vi "MU Calibration Get Nonius Track Offset Table.vi"(8 "error in (no error)":errorcluster, 11 "CalibrationHandle":T1) -> (0 "error out (no error)":errorcluster, 3 "noniusTrackOffsetTable":cluster{"spoBase":i8, "spoN":i8[]})   [LabVIEW 2017, in "MU_3SL_interface.lvlib"]
uses:
  MU_3SL_interface.lvlib
  handles/CalibrationHandle.ctl
  lib/MU_3SL_interface.dll
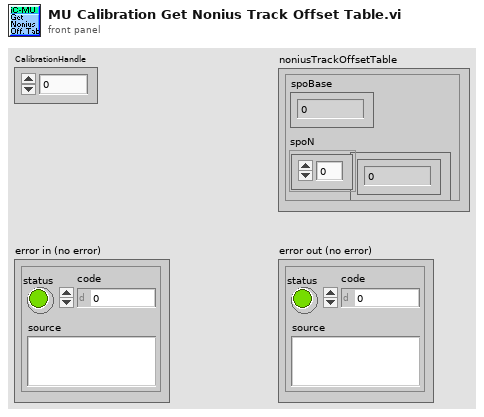
[diagram p1: front panel]
types:
  T1 = typedef "MU_3SL_interface.lvlib/CalibrationHandle.ctl" = u64
  T2 = cluster{"[0]":i8, "[1]":i8, "[2]":i8, "[3]":i8, "[4]":i8, "[5]":i8, "[6]":i8, "[7]":i8, "[8]":i8, "[9]":i8, "[10]":i8, "[11]":i8, "[12]":i8, "[13]":i8, "[14]":i8, "[15]":i8, "[16]":i8}
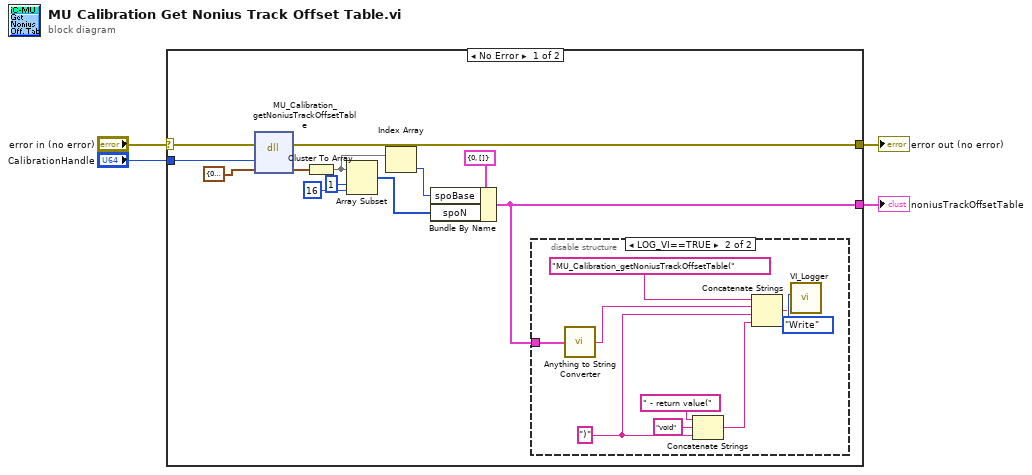
[diagram p0: block diagram]
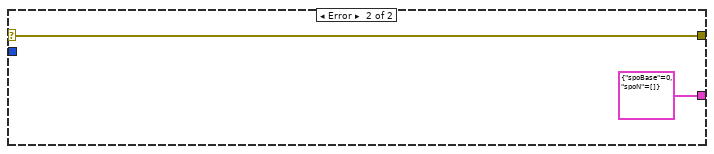
[diagram p3: hidden frame]
diagram:
  n1 = case shown="No Error" "error in (no error)" {
    selector: "error in (no error)" -> [w16 w27]
    tunnel: [w14 w27] -> w4
    tunnel: "CalibrationHandle" -> [w15 _]
    tunnel: [w5 cluster{"spoBase":i8, "spoN":i8[]} {"spoBase"=0, "spoN"=[]} ("optimizedNoniusTrackOffsetTable")] -> w2
    frame No Error {
      n2 = dll-call lib="C:/Users/bes/AppData/Roaming/work/mu_9so/icsubmodules/soft_mu_3sl_master/lv_interface/lib/MU_3SL_interface**.*" fn="MU_Calibration_getNoniusTrackOffsetTable"(error in=w16, "CalibrationHandle"=w15, "noniusTrackOffsetTable"=T2 {"[0]"=0, "[1]"=0, "[2]"=0, "[3]"=0, "[4]"=0, "[5]"=0, "[6]"=0, "[7]"=0, "[8]"=0, "[9]"=0, "[10]"=0, "[11]"=0, "[12]"=0, "[13]"=0, "[14]"=0, "[15]"=0, "[16]"=0}) -> (error out=w14:errorcluster, "noniusTrackOffsetTable"=w8:T2)  [unwired: 4 in, 1 out]
      n3 = Cluster To Array(cluster=w8) -> (array=w11:i8[])
      n4 = Array Subset(array=w11, index=1, length=16) -> (w9:i8[])
      n5 = Index Array(array=w11) -> (element=w10:i8)  [unwired: 1 in]
      n6 = Bundle By Name(cluster=cluster{"spoBase":i8, "spoN":i8[]} {"spoBase"=0, "spoN"=[]} ("optimizedNoniusTrackOffsetTable"), "spoBase"=w10, "spoN"=w9) -> (w5:cluster{"spoBase":i8, "spoN":i8[]})
      n7 = disable-structure shown="LOG_VI==TRUE" {
        disable-tunnel: w5 -> [_ w20]
        frame condition #0 {
        }
        frame condition #1 (active) {
          w19 = ")" ("string")
          n8 = call "Anything to String Converter.vi"("anything"=w20) -> ("String"=w18:string)
          n9 = Concatenate Strings(" - return value(" ("string"), "void" ("string"), w19) -> (w17:string)
          n10 = Concatenate Strings("MU_Calibration_getNoniusTrackOffsetTable(" ("Info in"), w18, w19, w17) -> (w23:string)
          n11 = call "VI_Logger.vi"("Action (Read)"=enum16{"Write", "Read"}."Write", "Info in"=w23) -> ()  [unwired: 8 in, 2 out]
        }
      }
    }
    frame Error {
    }
  }
  "error out (no error)" <- w4
  "noniusTrackOffsetTable" <- w2
